vi "Digital Read Pulse Width.vi"(5 "Incoming Pulse Polarity (Active High)":T2=enum."Active High", 6 "Timeout  (250 mS)":u32=250, 7 "Stimulus Pulse (Active High)":T1=enum."Active High", 8 "Error In":errorcluster={"status"=FALSE, "code"=1073676294, "source"="VISA Read in LVH-LINX.lvlib:Device.lvlib:Serial Read.vi->LVH-LINX.lvlib:Device.lvlib:Wait For Packet.vi->LVH-LINX.lvlib:Device.lvlib:Send Command.vi->LVH-LINX.lvlib:Device.lvlib:Digital Read Pulse Width.vi->Untitled 5"}, 9 "DO Channel (0)":u8, 10 "DI Channel (0)":u8=8, 11 "LINX Device Config":T3={"Interface"=enum."Serial", "COM Port"="COM5", "TCP Configuration"={"IP Address"="", "Port"=0}, "Device Family"=1, "Device ID"=1, "Device Name"="chipKIT uC32", "TCP Ref"=refnum, "Channels"={"DI"=[], "DO"=[], "AI"=[], "AO"=[], "PWM"=[], "QE"=[], "UART"=[], "I2C 2"=[], "SPI"=[], "CAN"=[], "Servo"=[], "AI Ref (V)"=0.0, "AI Resolution (Bits)"=0, "AO Ref (V)"=0.0, "AO Resolution (Bits)"=0}}) -> (0 "Error Out":errorcluster={"status"=FALSE, "code"=1073676294, "source"="VISA Read in LVH-LINX.lvlib:Device.lvlib:Serial Read.vi->LVH-LINX.lvlib:Device.lvlib:Wait For Packet.vi->LVH-LINX.lvlib:Device.lvlib:Send Command.vi->LVH-LINX.lvlib:Device.lvlib:Digital Read Pulse Width.vi->Untitled 5"}, 2 "Pulse Width (uS)":u32, 3 "LINX Device Config":T3={"Interface"=enum."Serial", "COM Port"="COM5", "TCP Configuration"={"IP Address"="", "Port"=0}, "Device Family"=1, "Device ID"=1, "Device Name"="chipKIT uC32", "TCP Ref"=refnum, "Channels"={"DI"=[], "DO"=[], "AI"=[], "AO"=[], "PWM"=[], "QE"=[], "UART"=[], "I2C 2"=[], "SPI"=[], "CAN"=[], "Servo"=[], "AI Ref (V)"=0.0, "AI Resolution (Bits)"=0, "AO Ref (V)"=0.0, "AO Resolution (Bits)"=0}})   [LabVIEW 2020, in "LMH-LINX.lvlib" / "Device.lvlib"]
uses:
  Device.lvlib
  Type Defs/LINX Device Config.ctl
  Type Defs/Interface.ctl
  Type Defs/TCP Config.ctl
  Type Defs/Channels.ctl
  Type Defs/Pulse Polarity.ctl
  Type Defs/Stimulus Pulse.ctl
  Type Defs/Error Type.ctl
  LMH-LINX.lvlib
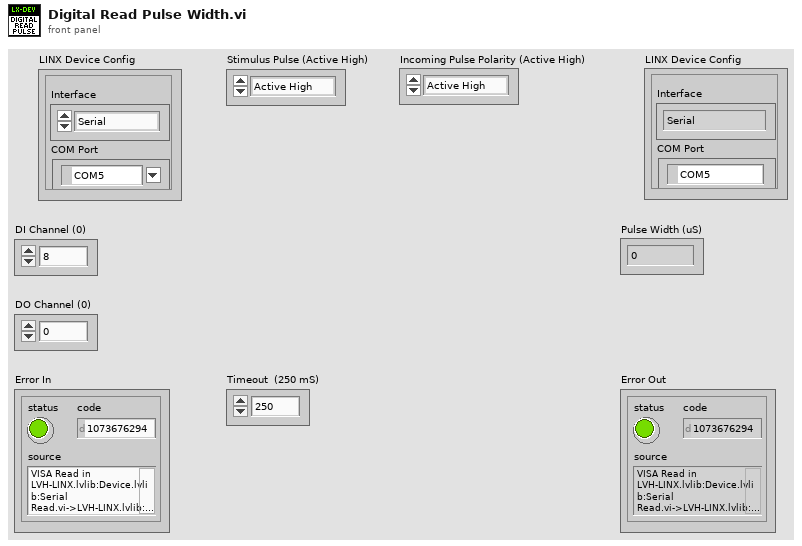
[diagram p1: front panel]
types:
  T1 = typedef "LMH-LINX.lvlib/Device.lvlib/Stimulus Pulse.ctl" = enum16{"None", "Active Low", "Active High"}
  T2 = typedef "LMH-LINX.lvlib/Device.lvlib/Pulse Polarity.ctl" = enum8{"Active Low", "Active High"}
  T3 = typedef "LMH-LINX.lvlib/Device.lvlib/LINX Device Config.ctl" = cluster{"Interface":T4, "COM Port":refnum<visa-resource-name>, "TCP Configuration":T5, "Device Family":u8, "Device ID":u8, "Device Name":string, "TCP Ref":refnum<k5>, "Channels":T6}
  T4 = typedef "LMH-LINX.lvlib/Interface.ctl" = enum16{"Serial", "TCP"}
  T5 = typedef "LMH-LINX.lvlib/Device.lvlib/TCP Config.ctl" = cluster{"IP Address":string, "Port":u16}
  T6 = typedef "LMH-LINX.lvlib/Channels.ctl" = cluster{"DI":u8[], "DO":u8[], "AI":u8[], "AO":u8[], "PWM":u8[], "QE":u8[], "UART":u8[], "I2C 2":u8[], "SPI":u8[], "CAN":u8[], "Servo":u8[], "AI Ref (V)":dbl, "AI Resolution (Bits)":u8, "AO Ref (V)":dbl, "AO Resolution (Bits)":u8}
  T7 = typedef "LMH-LINX.lvlib/Error Type.ctl" = enum16{"Unknown", "Timeout", "Corrupt Return Packet", "Unable To Connect", "Command Not Supported", "Channel DNE", "Invalid COM Config", "Firmware Version Mismatch", "myRIO Support", "CMD Specific Error", "Local IO Not Supported"}
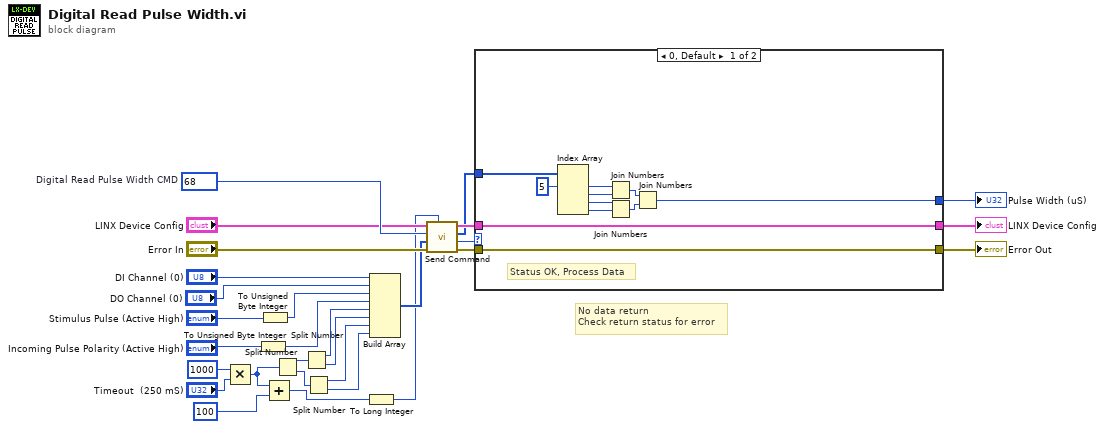
[diagram p0: block diagram]
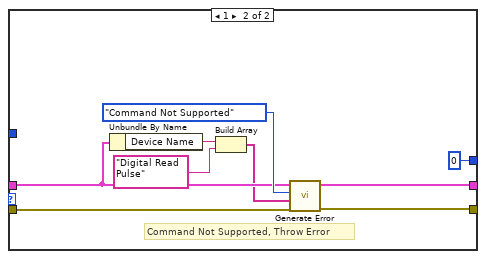
[diagram p2: hidden frame]
diagram:
  w28 = u16 68  # Digital Read Pulse Width CMD
  # "No data return\nCheck return status for error"
  n1 = Multiply(x=u32 1000 ("y"), y="Timeout  (250 mS)") -> (x*y=w7:u32)
  n2 = To Unsigned Byte Integer(number="Incoming Pulse Polarity (Active High)") -> (unsigned 8bit integer=w20:u8)
  n3 = To Unsigned Byte Integer(number="Stimulus Pulse (Active High)") -> (unsigned 8bit integer=w22:u8)
  n4 = Add(x=w7, y=u32 100) -> (x+y=w2:u32)
  n5 = Split Number(x=w7) -> (hi(x)=w18:u16, lo(x)=w17:u16)
  n6 = Split Number(x=w18) -> (hi(x)=w16:u8, lo(x)=w15:u8)
  n7 = Split Number(x=w17) -> (hi(x)=w14:u8, lo(x)=w13:u8)
  n8 = To Long Integer(number=w2) -> (32bit integer=w1:i32)
  n9 = Build Array("DI Channel (0)", "DO Channel (0)", w22, w20, w16, w15, w14, w13) -> (w12:u8[])
  n10 = call "Send Command.vi"("Timeout (100 ms)"=w1, "Error In"="Error In", "ARGS"=w12, "CMD"=w28, "LINX Device Config"="LINX Device Config") -> ("Error Out"=w23:errorcluster, "Status"=w11:u8, "Response"=w10:u8[], "LINX Device Config"=w25:T3)  [unwired: 3 in]
  n11 = case shown="0, Default" w11 {
    tunnel: [w40 w47] -> w26
    tunnel: w25 -> [w40 w43]
    tunnel: [w39 w48] -> w24
    tunnel: w23 -> [w39 w49]
    tunnel: w10 -> [w38 _]
    tunnel: [w30 u32 0] -> w9
    frame 0, Default {
      # "Status OK, Process Data"
      n12 = Index Array(array=w38, index #1=5 ("index")) -> (element #1=w36:u8, element #2=w35:u8, element #3=w34:u8, element #4=w33:u8)  [unwired: 3 in]
      n13 = Join Numbers(hi=w36, lo=w35) -> ((hi.lo)=w32:u16)
      n14 = Join Numbers(hi=w34, lo=w33) -> ((hi.lo)=w31:u16)
      n15 = Join Numbers(hi=w32, lo=w31) -> ((hi.lo)=w30:u32)
    }
    frame 1 {
      # "Command Not Supported, Throw Error"
      n16 = Unbundle By Name(w43) -> ("Device Name"=w45:string)
      n17 = Build Array(w45, "Digital Read Pulse") -> (w42:string[])
      n18 = call "Generate Error.vi"("Error In"=w49, "Arguments"=w42, "Error Type"=Error_Type."Command Not Supported", "LINX Device Config"=w43) -> ("Error Out"=w48:errorcluster, "Dup LINX Device Config"=w47:T3)  [unwired: 6 in]
    }
  }
  "Error Out" <- w24
  "LINX Device Config" <- w26
  "Pulse Width (uS)" <- w9
